vi "motor init.vi"(5 "encoder":cluster{"encoder PPR":dbl, "gear ratio":dbl}, 6 "motor  ?":enum16{"M1", "M2", "M3", "M4"}(ring), 7 "dt":dbl, 8 "Error In":errorcluster, 9 "PWM frequence":dbl, 10 "PID":cluster{"Kp":dbl, "Ki":dbl, "Kd":dbl}, 11 "class in":refnum<class "motor.lvclass">) -> (0 "error out":errorcluster, 3 "class out":refnum<class "motor.lvclass">)   [LabVIEW 2019, in "my FPGA lib.lvlib" / "motor.lvclass"]
uses:
  motor.lvclass
  motor.lvclass/motor.ctl
  my FPGA lib.lvlib
panel:
  in  "V.PID Path":path=path "C:/Users/robot/Desktop/Labview/smallmom-3/FPGA_subVIs/low level/motor/math/PID.vi"
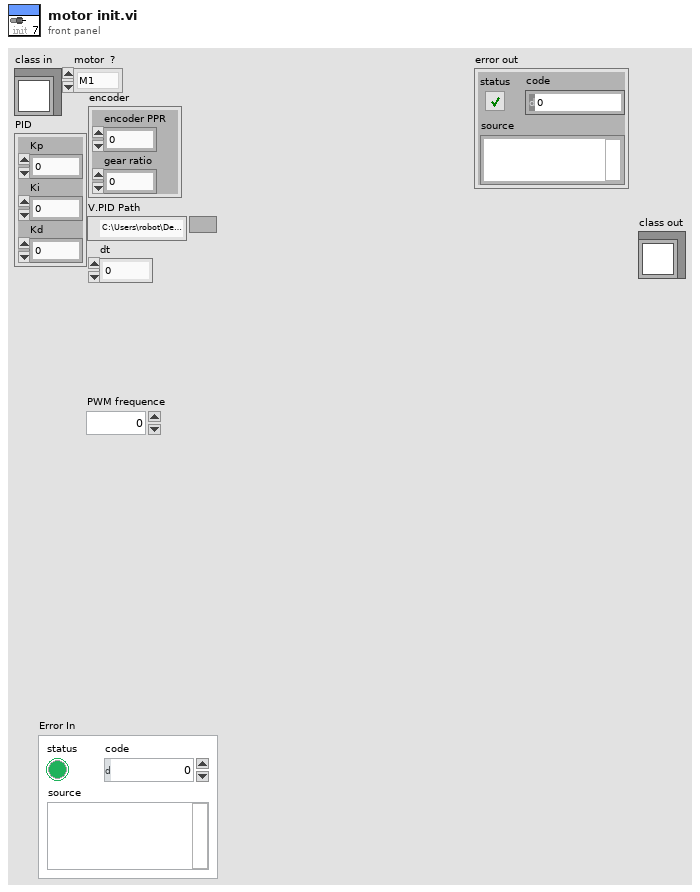
[diagram p1: front panel]
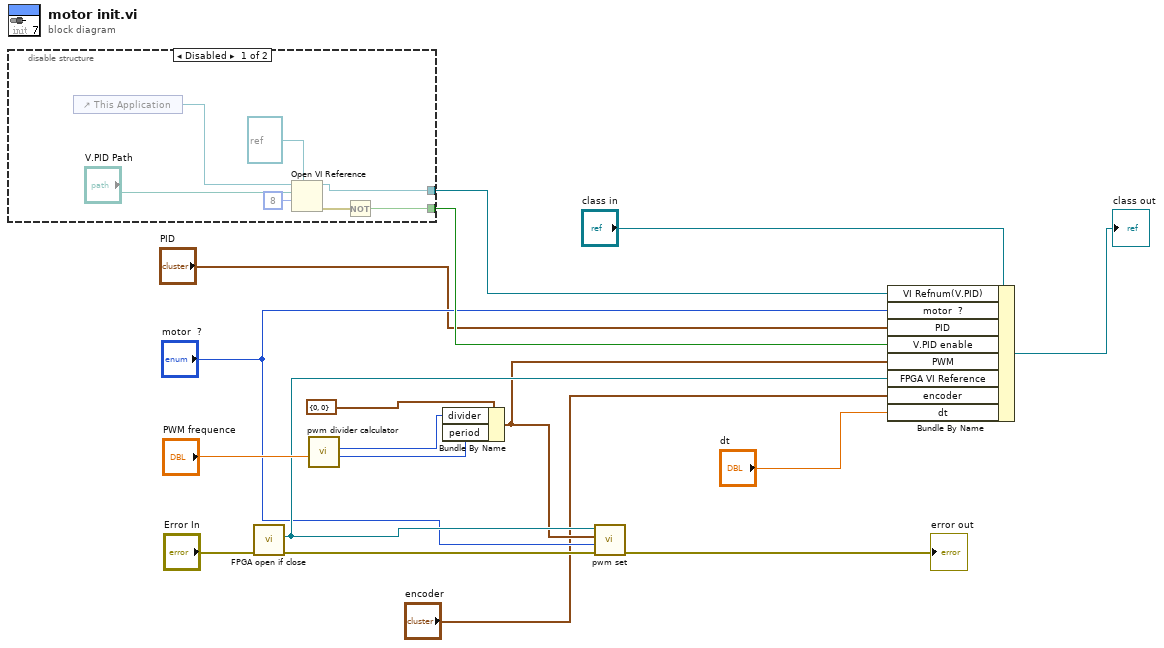
[diagram p0: block diagram]
diagram:
  n1 = disable-structure shown="Disabled" {
    disable-tunnel: [w24 _] -> w14
    disable-tunnel: [w23 _] -> w3
    frame Disabled {
      n2 = control-ref of="This Application"() -> (w19:refnum<vi>)
      n3 = Open VI Reference(type specifier VI Refnum (for type only)=refnum<vi> refnum, application reference (local)=w19, vi path="V.PID Path", options=8) -> (vi reference=w23:refnum<vi>, error out=w18:errorcluster)  [unwired: 2 in]
      n4 = Not(x=w18) -> (.not. x?=w24:bool)
    }
    frame Enabled {
    }
  }
  n5 = call "FPGA open if close.vi"("error in"="Error In") -> ("error out"=w9:errorcluster, "FPGA VI Reference Out"=w8:refnum<k20>)  [unwired: 9 in]
  n6 = call "pwm divider calculator.vi"("PWM frequence"="PWM frequence") -> ("period"=w10:i32, "divider rate"=w11:i32)  [unwired: 6 in, 1 out]
  n7 = Bundle By Name(cluster=cluster{"divider":i32, "period":i32} {"divider"=0, "period"=0} ("PWM"), "divider"=w11, "period"=w10) -> (w7:cluster{"divider":i32, "period":i32})
  n8 = call "pwm set.vi"("error in"=w9, "motor  ?"="motor  ?", "PWM"=w7, "FPGA VI Reference In"=w8) -> ("error out"=→"error out":errorcluster)  [unwired: 6 in, 1 out]
  n9 = Bundle By Name(cluster="class in", "VI Refnum(V.PID)"=w3, "motor  ?"="motor  ?", "PID"="PID", "V.PID enable"=w14, "PWM"=w7, "FPGA VI Reference"=w8, "encoder"="encoder", "dt"="dt") -> (→"class out":refnum<class "motor.lvclass">)
